vi "Práctica 1_Dídier Javier Ramírez Henao.vi"() -> ()   [LabVIEW 2020]
panel:
  in  "Marcha":bool
  in  "Paro":bool
  out "Almacenamiento Silo 1":i32(slide) scale=0.0..50.0
  # "Subproceso 1"
  # "Dídier Javier Ramírez Henao"
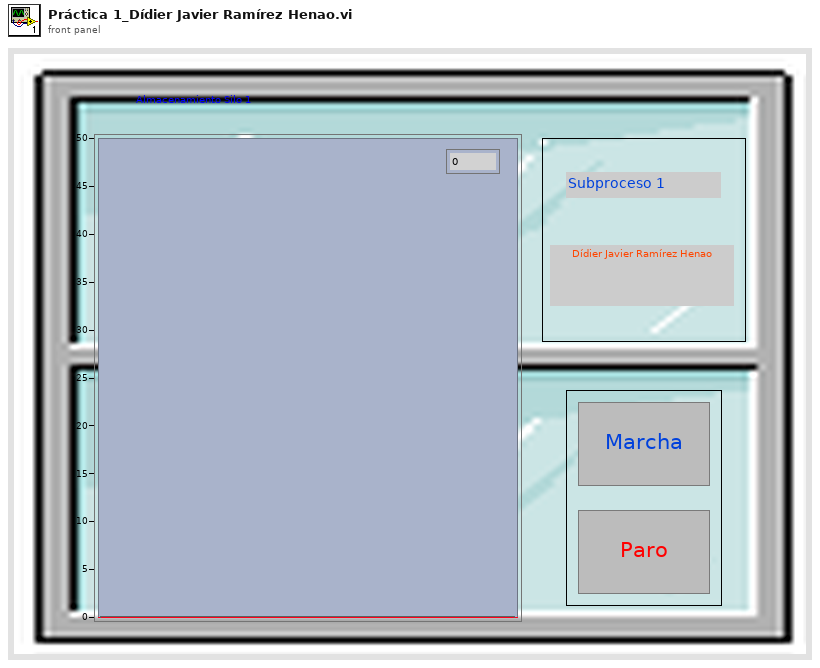
[diagram p1: front panel]
types:
  T1 = enum16{"INICIO", "INCREMENTO", "DECREMENTO", "FIN"}
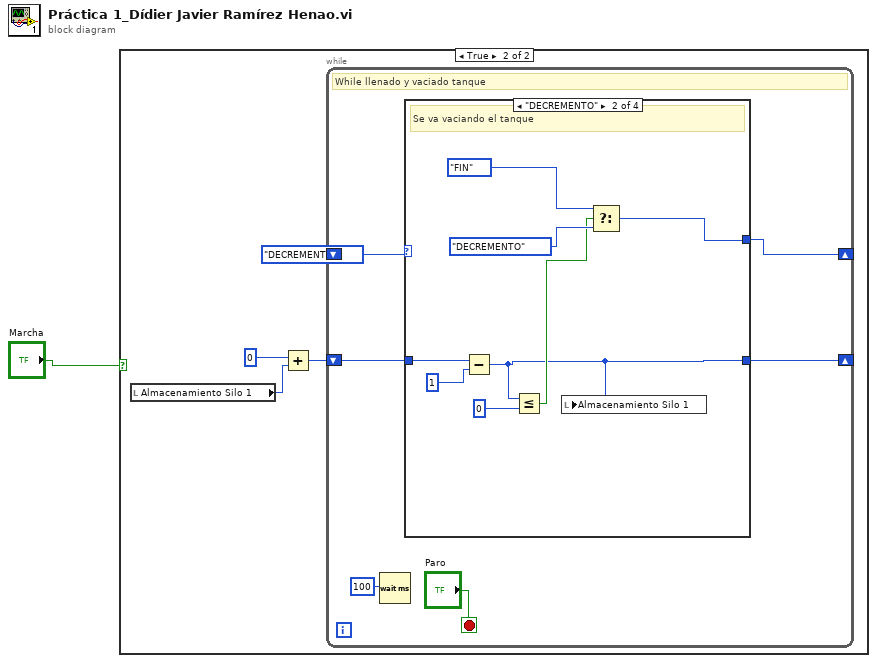
[diagram p0: block diagram]
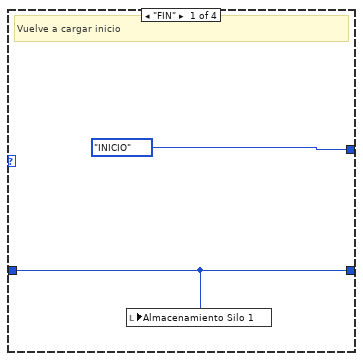
[diagram p3: hidden frame]
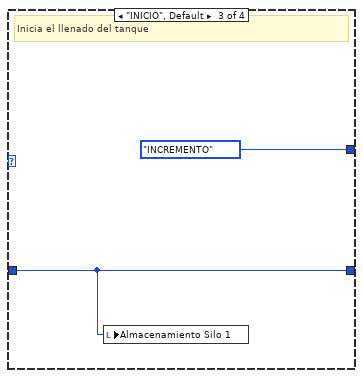
[diagram p4: hidden frame]
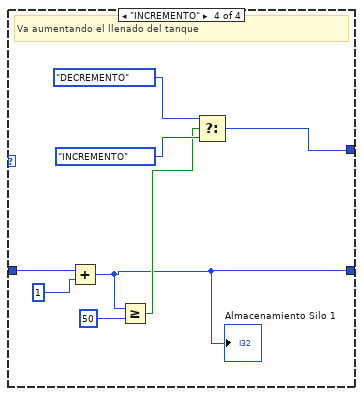
[diagram p5: hidden frame]
diagram:
  n1 = case shown="True" "Marcha" {
    frame False {
    }
    frame True {
      n2 = local read "Almacenamiento Silo 1"() -> (w2:i32)
      n3 = Add(x=0, y=w2) -> (x+y=w4:i32)
      n4 = while {
        shift-right: [w9] -> _
        shift-left: w4 -> [w10]
        shift-right: [w7] -> _
        shift-left: T1."DECREMENTO" -> [w8]
        stop <- "Paro" stop-if-true
        # "While llenado y vaciado tanque"
        n5 = Wait (ms)(milliseconds to wait=u32 100 ("millisecond timer value")) -> ()  [unwired: 1 out]
        n6 = case shown="\"DECREMENTO\"" w8 {
          tunnel: w10 -> [w13 w16 w23 w31]
          tunnel: [w13 w14 w23 w24] -> w9
          tunnel: [T1."INICIO" w15 T1."INCREMENTO" w27] -> w7
          frame "FIN" {
            # "Vuelve a cargar inicio"
            n7 = local write "Almacenamiento Silo 1"(w13) -> ()
          }
          frame "DECREMENTO" {
            # "Se va vaciando el tanque"
            n8 = Subtract(x=w16, y=1) -> (x-y=w14:i32)
            n9 = Less Or Equal?(x=w14, y=0) -> (x <= y?=w17:bool)
            n10 = local write "Almacenamiento Silo 1"(w14) -> ()
            n11 = Select(t=T1."FIN", s=w17, f=T1."DECREMENTO") -> (s? t:f=w15:T1)
          }
          frame "INICIO", Default {
            # "Inicia el llenado del tanque"
            n12 = local write "Almacenamiento Silo 1"(w23) -> ()
          }
          frame "INCREMENTO" {
            # "Va aumentando el llenado del tanque"
            n13 = Add(x=w31, y=1) -> (x+y=w24:i32)
            "Almacenamiento Silo 1" <- w24
            n14 = Greater Or Equal?(x=w24, y=50) -> (x >= y?=w25:bool)
            n15 = Select(t=T1."DECREMENTO", s=w25, f=T1."INCREMENTO") -> (s? t:f=w27:T1)
          }
        }
      }
    }
  }
